vi "RTU2Str.vi"(1 "RTU数据帧":u8[](array[numeric])) -> (0 "RTU数据帧字符串":string)   [LabVIEW 2015]
doc: "用于显示的带空格字符的RTU字符串"
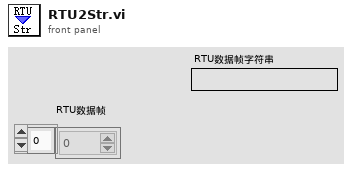
[diagram p1: front panel]
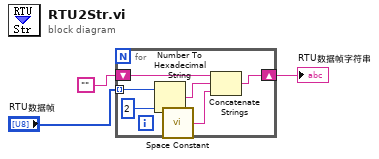
[diagram p0: block diagram]
diagram:
  n1 = for {
    tunnel: "RTU数据帧" -> [w9] mode=indexing
    shift-right: [w6] -> w1
    shift-left: "" -> [w7]
    n2 = Number To Hexadecimal String(1:2, 2:w9) -> (0:w8:string)
    n3 = call <vilib>:"Space Constant.vi"() -> ("String"=w4:string)
    n4 = Concatenate Strings(w7, w8, w4) -> (w6:string)
  }
  "RTU数据帧字符串" <- w1
